vi "RunTest.vi"(8 "error in (no error)":errorcluster, 11 "Prueba07 in":refnum<class "Prueba07.lvclass">) -> (0 "error out":errorcluster, 2 "resultado":string, 3 "Prueba07 out":refnum<class "Prueba07.lvclass">)   [LabVIEW 2019, in "Prueba07.lvclass"]
uses:
  Prueba07.lvclass
  Prueba04/Control/Slide.ctl
  Prueba07.lvclass/Prueba07.ctl
  ClusterGEN.ctl
  Controles/MessageP07.ctl
  Controles/EstadosP07.ctl
  <vilib>/Utility/error.llb/DialogType.ctl
  QMH/Message Queue/Enqueue Message (Single).vi
  <vilib>/Utility/error.llb/Error Cluster From Error Code.vi
  <vilib>/ErrorRing/Error Ring.xnode
  <vilib>/Utility/miscctls.llb/LVRowAndColumnTypeDef.ctl
  Prueba/Prueba.lvclass
  Prueba04/Prueba04.lvclass
  QMH/User Event - Stop/User Event - Stop.lvlib
  QMH/Message Queue/Message Queue.lvlib
panel:
  out "GEN":string
  out "n°filas":i32
  out "Vref_NivMax":dbl[](array[numeric])
  out "tablaRef (Num)":dbl[](array[numeric])
  out "Pict Ring 2":u16(ring)
  out "Pict Ring 3":u16(ring)
  out "cumple_no_cumple":bool
  out "Vref":dbl
  in  "Tab":enum32{"Page 1", "Page 2"}(tab)
  out "frecuencia1":dbl=140.0
  out "nivelRef":dbl=95.0 format="%.1f"
  in  "guardar_Vref":bool
  in  "generar1":bool
  in  "AjusteAmp":T1=50.0 caption="Ajuste de amplitud [mV]" scale=0.0..100.0
  out "voltaje1":dbl format="%.1f"
  out "frecuencia1":dbl format="%.1f"
  in  "seguir":bool
  out "Pict Ring 1":u16(ring)
  out "Pict Ring":u16(ring)
  out "RefActual":string
  in  "generarNivMax":bool caption="PruebaSup"
  in  "generarNivRef":bool caption="PruebaSup"
  in  "Tabla":string[][](table)
  in  "salir":bool
  out "cumple":bool
  out "no_cumple":bool
  out "voltaje2":dbl format="%.1f"
  out "frecuencia2":dbl format="%#.1f"
  out "RangoRefActual":string
  # "Elección Señal de Referencia\nsegún marca y modelo de sonómetro"
  # "Nivel Señal Referencia"
  # "Frecuencia"
  # "Monitoreo"
  # "Frecuencia"
  # "Hz"
  # "Voltaje"
  # "mV"
  # "7. Linealidad de nivel incluyendo el control de rangos de niveles. IEC 61672-3: 2006 Cláusula 15"
  # "Tabla Resultados"
  # "Nivel de Referencia"
  # "Nivel Max Rn - 5 db(A)"
  # "Rango dB"
  # "Referencia dB"
  # "Cumple"
  # "No Cumple"
  # "7. Linealidad de nivel incluyendo el control de rangos de niveles. IEC 61672-3: 2006 Cláusula 15"
  # "Monitoreo"
  # "Frecuencia"
  # "Hz"
  # "Voltaje"
  # "mV"
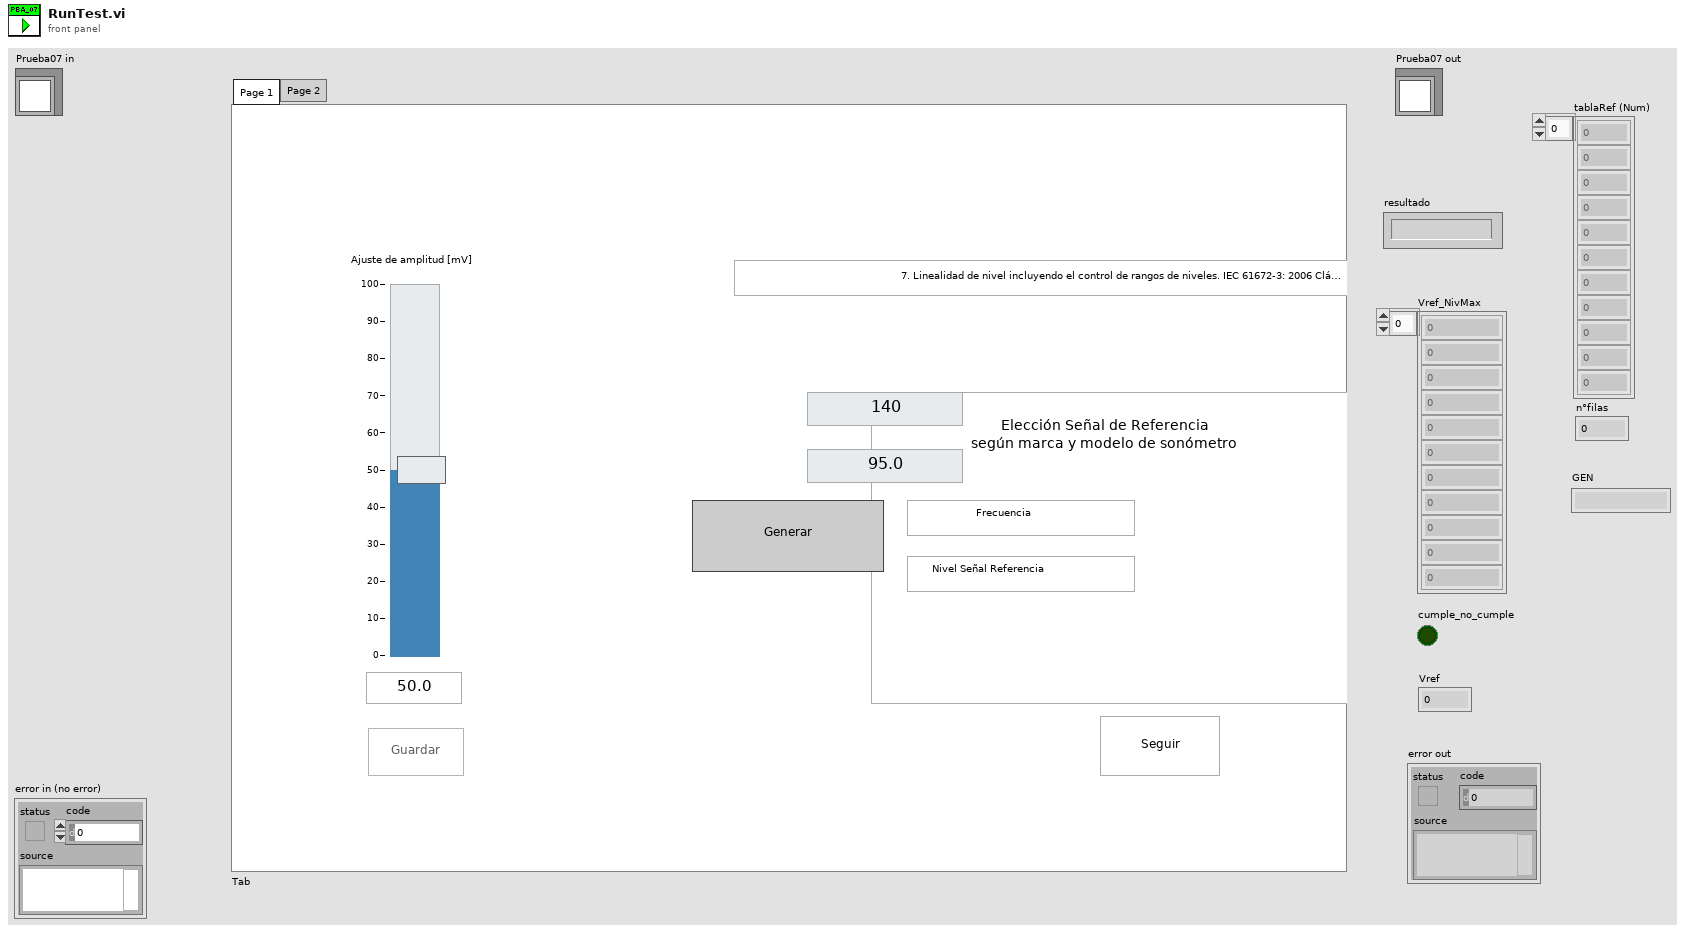
[diagram p1: front panel]
types:
  T1 = typedef "Prueba04.lvclass/Slide.ctl" = dbl
  T2 = typedef "LVRowAndColumnTypeDef.ctl" = cluster{"Row":i32, "Column":i32}
  T3 = typedef "Message Queue.lvlib/All Message Queues.ctl" = cluster{"MHL":refnum<queue>, "Inst_CNT90":refnum<queue>, "Inst_DS360":refnum<queue>, "Inst_Keithley2002":refnum<queue>, "Inst_DAQ":refnum<queue>, "BD":refnum<queue>, "Pistofono":refnum<queue>, "Nexus":refnum<queue>}
  T4 = enum32{"Page 1", "Page 2", "Page 3", "Page 4", "Page 5", "Page 6", "Page 7"}
  T5 = typedef "Prueba07.lvclass/ClusterGEN.ctl" = cluster{"frec":dbl, "amp":dbl}
  T6 = enum8{"Enabled", "Disabled", "Disabled and Grayed Out"}
  T7 = cluster{"ControlName":string, "ControlReference":refnum<vi>}[]
  T8 = typedef "Prueba07.lvclass/MessageP07.ctl" = cluster{"Estados":T9, "Data":variant}
  T9 = typedef "Prueba07.lvclass/EstadosP07.ctl" = enum16{"inicio", "LeerArchivoConfiguracion", "InicializarInstrumentos", "DetieneInstrumentos", "leerRangosdB", "configuraTabla", "FrecAmp1", "FrecAmp2_Vref", "updateUI", "FrecAmp2_Vref_NivMax", "iniciarGEN", "detenerGEN", "guardaVref", "monitoreo", "calcular_Vref", "guardarMedicionesNivRef", "guardarMedicionesNivMax", "ingresaMediciones", "cumplimiento", "listo_evaluar", "evaluar", "final", "salir"}
  T10 = typedef "DialogType.ctl" = u16
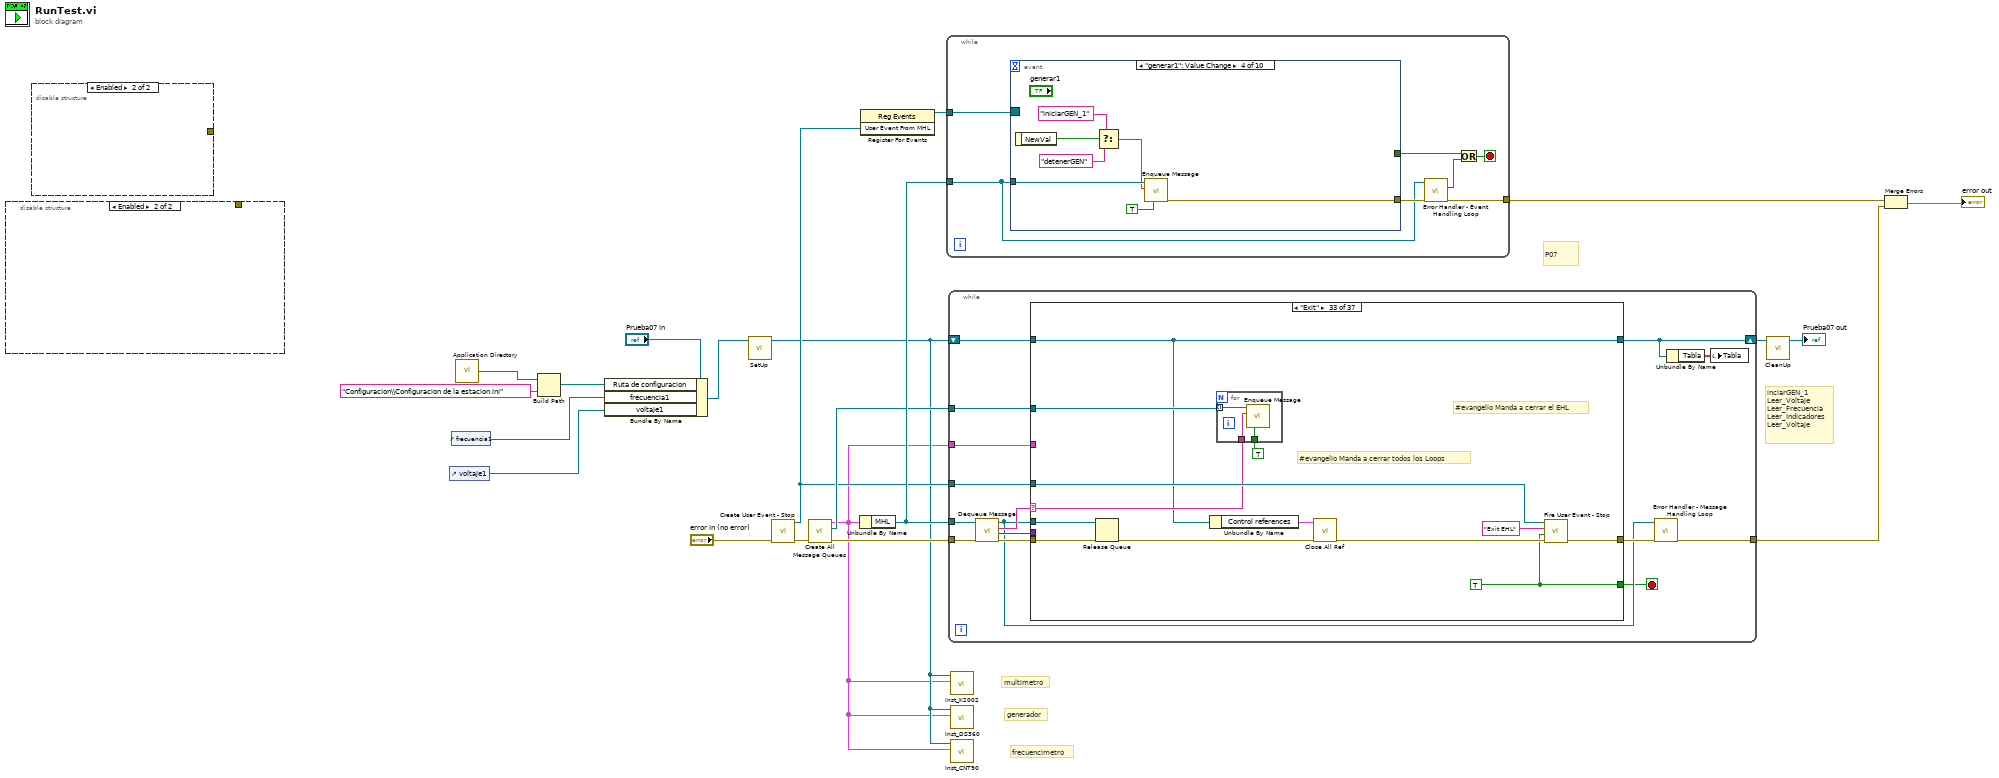
[diagram p0: block diagram]
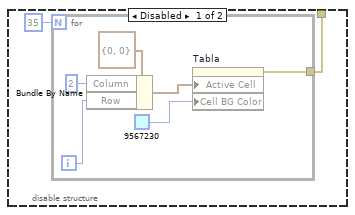
[diagram p2: hidden frame]
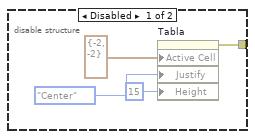
[diagram p3: hidden frame]
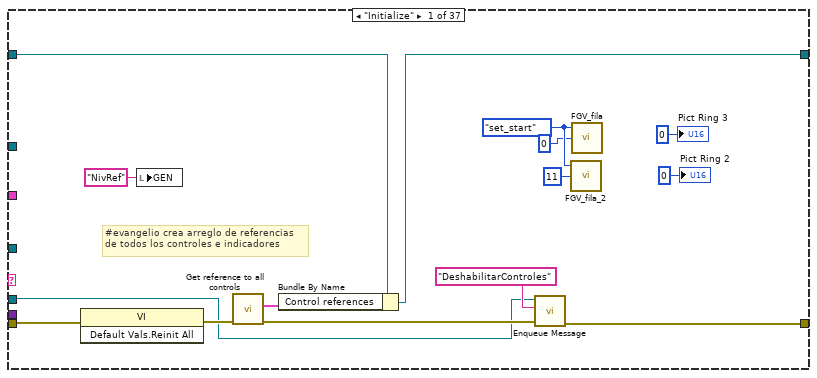
[diagram p4: hidden frame]
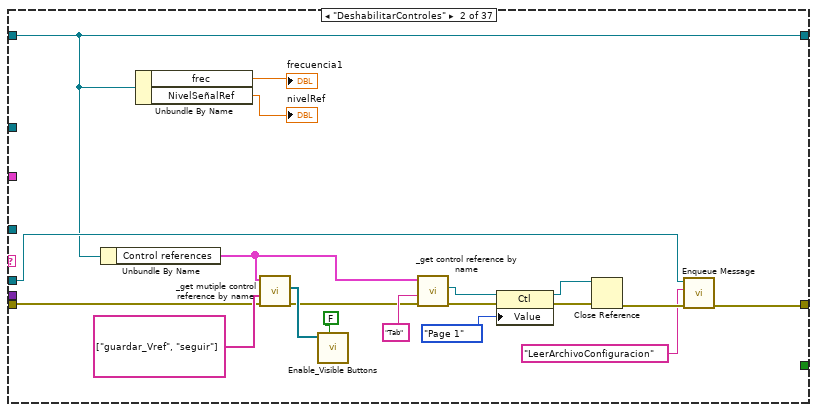
[diagram p5: hidden frame]
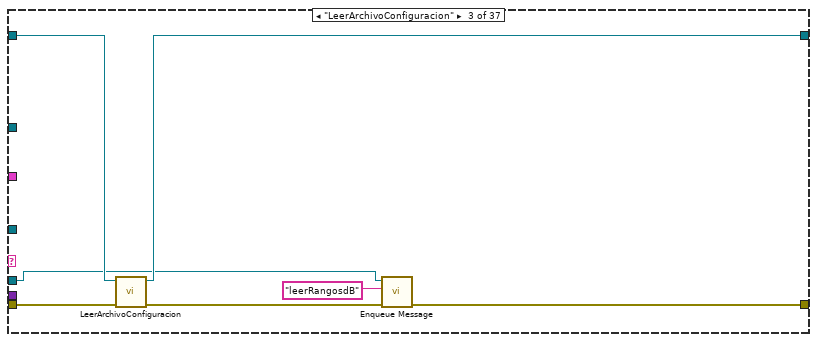
[diagram p6: hidden frame]
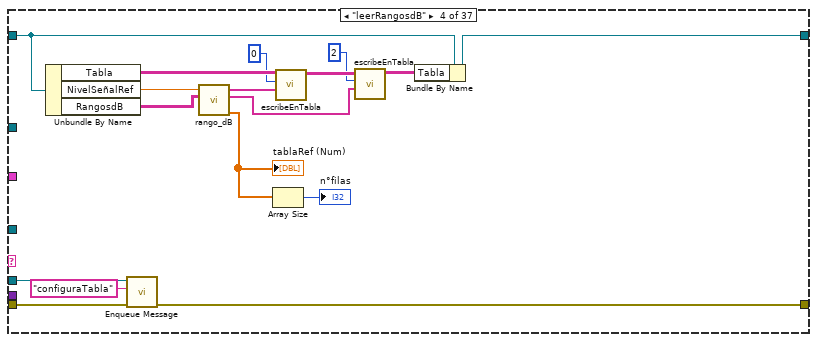
[diagram p7: hidden frame]
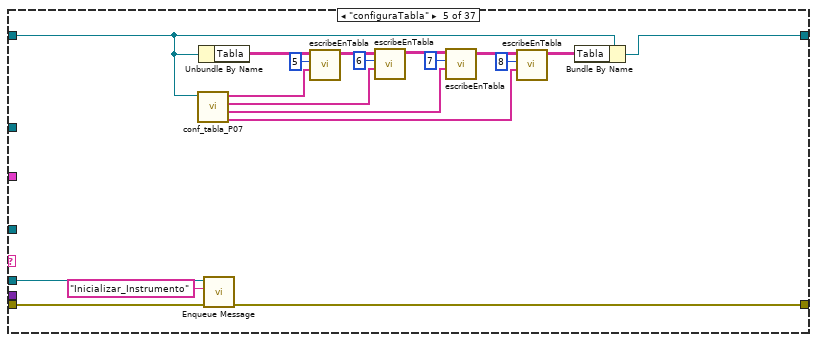
[diagram p8: hidden frame]
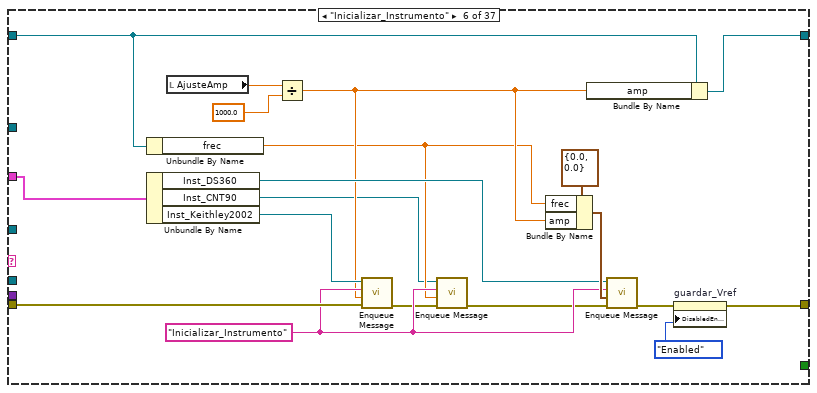
[diagram p9: hidden frame]
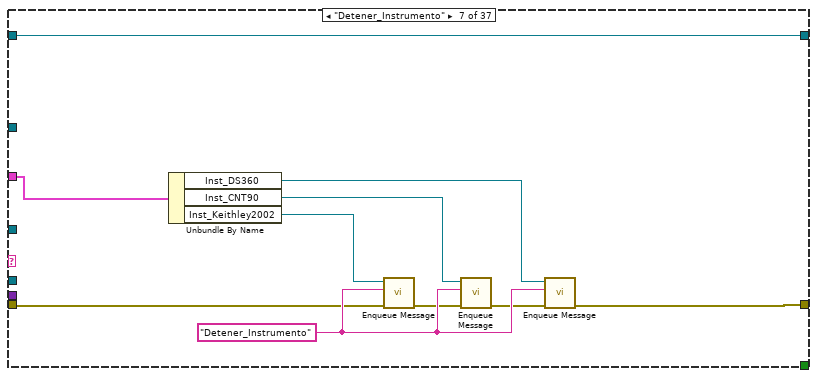
[diagram p10: hidden frame]
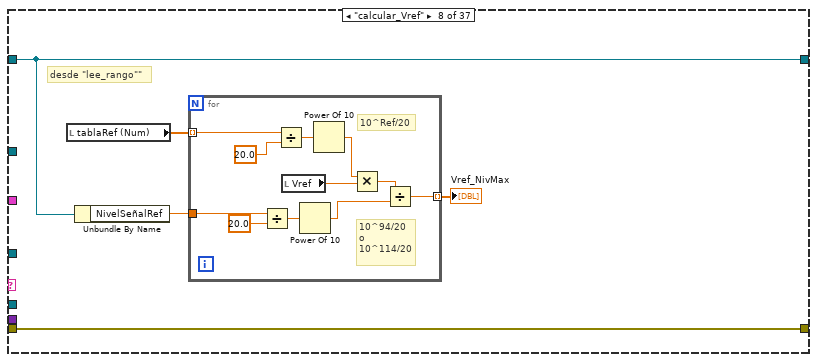
[diagram p11: hidden frame]
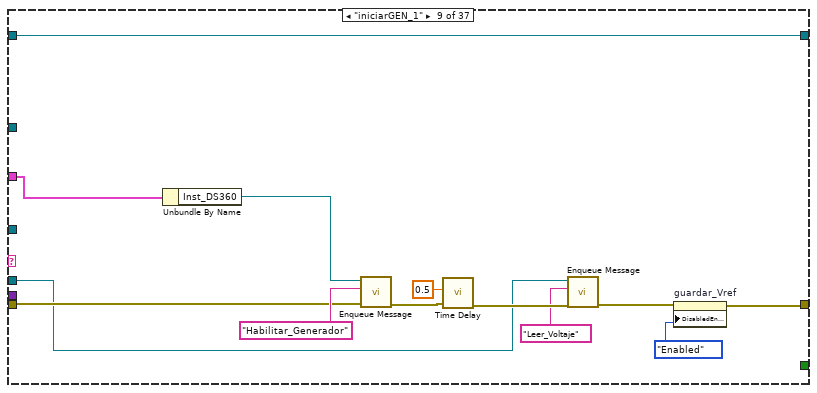
[diagram p12: hidden frame]
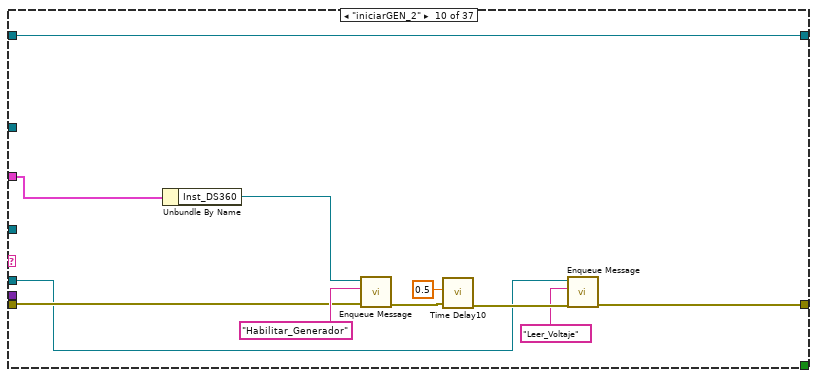
[diagram p13: hidden frame]
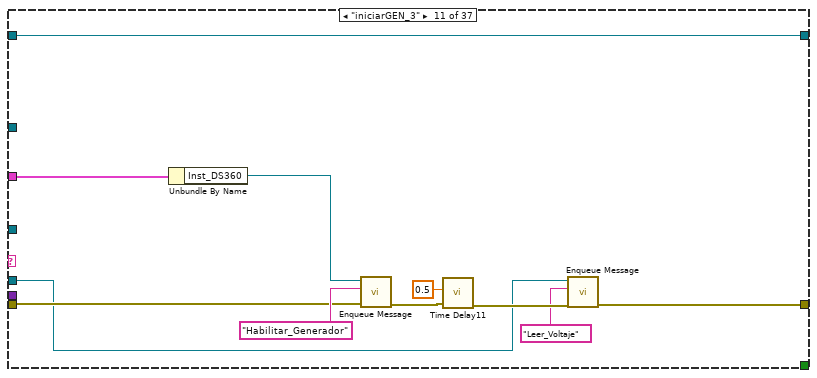
[diagram p14: hidden frame]
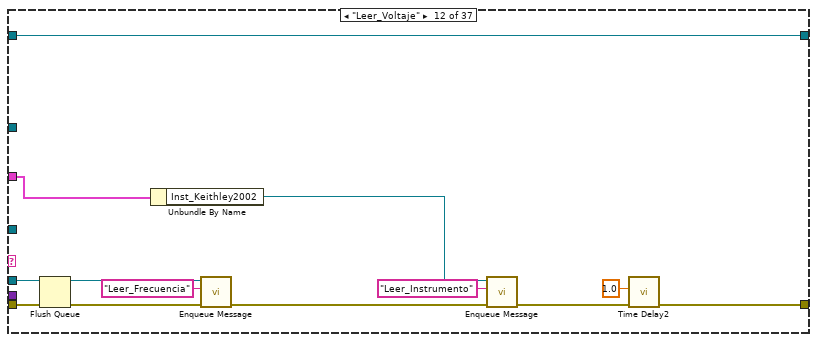
[diagram p15: hidden frame]
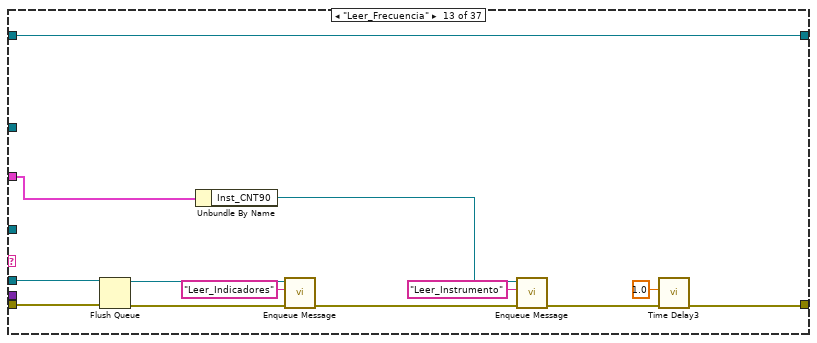
[diagram p16: hidden frame]
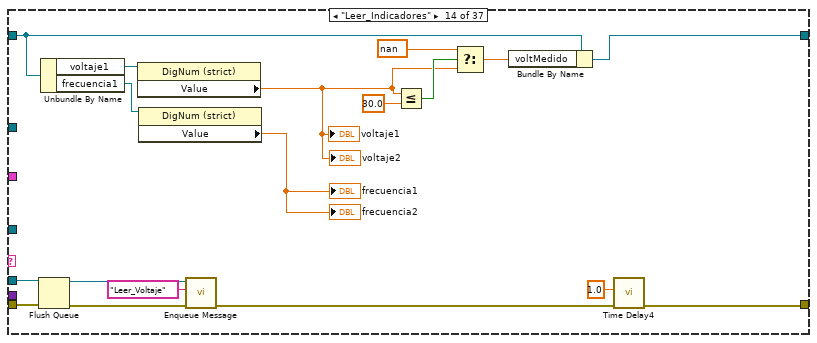
[diagram p17: hidden frame]
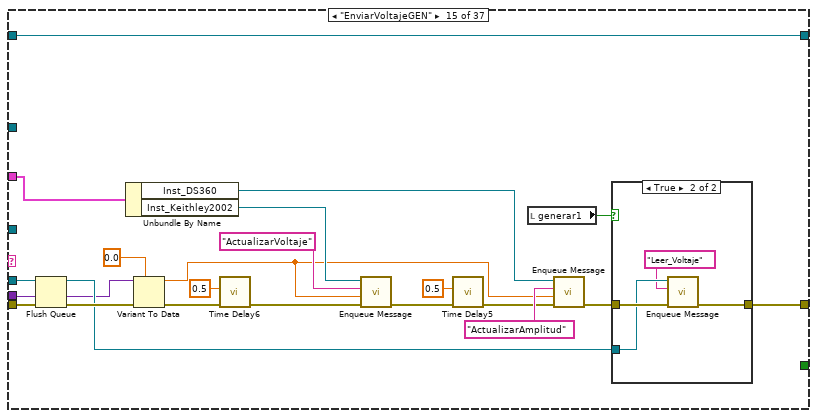
[diagram p18: hidden frame]
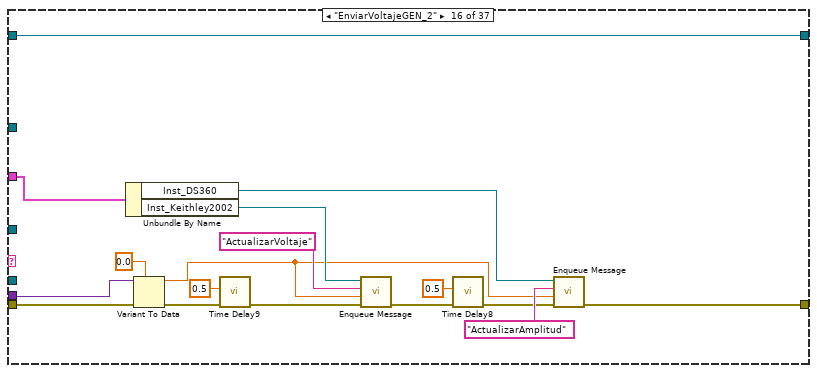
[diagram p20: hidden frame]
diagram:
  # "inciarGEN_1\nLeer_Voltaje\nLeer_Frecuencia\nLeer_Indicadores\nLeer_Voltaje"
  # "P07"
  # "frecuencimetro"
  # "generador"
  # "multimetro"
  n1 = disable-structure shown="Enabled" {
    disable-tunnel: [w23 _] -> _
    frame Disabled {
      n2 = for {
        N: 35 -> [_]
        tunnel: [w25] -> w23
        i -> [w24]
        n3 = Bundle By Name(cluster=T2 {"Row"=0, "Column"=0} ("Active Cell:Active Cell"), "Column"=2, "Row"=w24) -> (w27:T2)
        n4 = property on="Tabla" class="Tbl (strict)"("Active Cell"=w27, "Cell BG Color"=u32 9567230) -> (error out=w25:errorcluster)  [unwired: 2 in, 1 out]
      }
    }
    frame Enabled {
    }
  }
  n5 = disable-structure shown="Enabled" {
    disable-tunnel: [w32 _] -> _
    frame Disabled {
      n6 = property on="Tabla" class="Tbl (strict)"("Active Cell"=T2 {"Row"=-2, "Column"=-2} ("Active Cell:Active Cell"), "Justify"=enum16{"Left", "Center", "Right"}."Center" ("Active Cell:Cell Justification"), "Height"=u32 15 ("Active Cell:Cell Font:Size")) -> (error out=w32:errorcluster)  [unwired: 2 in, 1 out]
    }
    frame Enabled {
    }
  }
  n7 = control-ref of="voltaje1"() -> (w3:refnum<vi>)
  n8 = control-ref of="frecuencia1"() -> (w4:refnum<vi>)
  n9 = call <vilib>:"Application Directory.vi"() -> ("Application Directory"=w17:path)
  n10 = Build Path(base path=w17, name or relative path="Configuracion\\Configuracion de la estacion.ini") -> (appended path=w16:path)
  n11 = Bundle By Name(cluster="Prueba07 in", "Ruta de configuracion"=w16, "frecuencia1"=w4, "voltaje1"=w3) -> (w14:refnum<class "Prueba07.lvclass">)
  n12 = call-dynamic "SetUp.vi"("Prueba07 in"=w14) -> ("Prueba07 out"=w6:refnum<class "Prueba07.lvclass">)  [unwired: 9 in, 1 out]
  n13 = call "Create User Event - Stop.vi"("error in (no error)"="error in (no error)") -> ("error out"=w13:errorcluster, "User Event From MHL"=w8:refnum<user-event>)  [unwired: 9 in]
  n14 = call "Create All Message Queues.vi"("error in (no error)"=w13) -> ("error out"=w11:errorcluster, "PL Queues Array"=w9:refnum<queue>[], "All Message Queues out"=w5:T3)  [unwired: 8 in]
  n15 = Unbundle By Name(w5) -> ("MHL"=w10:refnum<queue>)
  n16 = register-events(w8) -> (reference out=w7:refnum<event-registration>)  [unwired: 2 in, 1 out]
  n17 = while {
    tunnel: w10 -> [w36]
    tunnel: [w38] -> w21
    tunnel: w7 -> [w35]
    stop <- w40 stop-if-true
    n18 = event shown="[3] \"generar1\": Value Change" {
      selector: w35 -> [_ _ _ _ _ _ _ _ _ _]
      dyn-events: _ -> [_ _ _ _ _ _ _ _ _ _]
      timeout: _ -> [_ _ _ _ _ _ _ _ _ _]
      tunnel: w36 -> [w43 _ w54 w61 w68 w75 w81 w87 w91 w97]
      tunnel: [w46 _ _ w62 w69 w76 w78 w88 w92 w96] -> w39
      tunnel: [_ w47 _ _ _ _ _ _ _ _] -> w34
      event "salir": Value Change {
        n19 = event-data() -> ()  [unwired: 1 in, 1 out]
        n20 = call-poly "Enqueue Message.vi"("Message"="Detener_Instrumento", "Message Queue"=w43) -> ("error out"=w41:errorcluster, "dup Message Queue"=w42:refnum<queue>)  [unwired: 8 in]
        n21 = call-poly "Enqueue Message.vi"("error in (no error)"=w41, "Message"="Exit", "Message Queue"=w42) -> ("error out"=w46:errorcluster)  [unwired: 7 in, 1 out]
      }
      event User Event {
        n22 = event-data() -> ("User Event"=w49:string, "Event Data"=w48:variant)  [unwired: 1 in]
        n23 = case shown="\"Exit EHL\"" w49 {
          tunnel: w48 -> [_ w51]
          tunnel: [_ w50] -> w47
          frame Default {
          }
          frame "Exit EHL" {
            # "#evangelio Termina\nla ejecucion del EHL"
            n24 = Variant To Data(type=TRUE, Variant=w51) -> (data=w50:bool)  [unwired: 1 in, 1 out]
          }
        }
      }
      event Panel Close? {
        w53 = TRUE
        n25 = event-data() -> ()  [unwired: 1 in, 1 out]
        n26 = call-poly "Enqueue Message.vi"("Priority Message? (F)"=w53, "Message"="Confirmar Salida", "Message Queue"=w54) -> ()  [unwired: 7 in, 2 out]
        n27 = event-data("Discard?"=w53) -> ()  [unwired: 1 in, 1 out]
      }
      event "generar1": Value Change {
        n28 = event-data() -> ("NewVal"=w60:bool)  [unwired: 1 in]
        n29 = Select(t="iniciarGEN_1" ("Message"), s=w60, f="detenerGEN" ("Message")) -> (s? t:f=w57:string)
        n30 = call-poly "Enqueue Message.vi"("Priority Message? (F)"=TRUE, "Message"=w57, "Message Queue"=w61) -> ("error out"=w62:errorcluster)  [unwired: 7 in, 1 out]
      }
      event "generarNivRef": Value Change {
        n31 = event-data() -> ("NewVal"=w67:bool)  [unwired: 1 in]
        n32 = Select(t="FrecAmp2_Vref", s=w67, f="guardarMedicionesNivRef") -> (s? t:f=w64:string)
        n33 = call-poly "Enqueue Message.vi"("Priority Message? (F)"=TRUE, "Message"=w64, "Message Queue"=w68) -> ("error out"=w69:errorcluster)  [unwired: 7 in, 1 out]
      }
      event "generarNivMax": Value Change {
        n34 = event-data() -> ("NewVal"=w74:bool)  [unwired: 1 in]
        n35 = Select(t="FrecAmp2_Vref_NivMax", s=w74, f="guardarMedicionesNivMax") -> (s? t:f=w71:string)
        n36 = call-poly "Enqueue Message.vi"("Priority Message? (F)"=TRUE, "Message"=w71, "Message Queue"=w75) -> ("error out"=w76:errorcluster)  [unwired: 7 in, 1 out]
      }
      event "seguir": Value Change {
        n37 = event-data() -> ()  [unwired: 1 in, 1 out]
        n38 = call-poly "Enqueue Message.vi"("Message"="calcular_Vref", "Message Queue"=w81) -> ("error out"=w79:errorcluster)  [unwired: 8 in, 1 out]
        n39 = property on="Tab" class="TabCtl (strict)"(error in=w79, "Value"=enum32{"Page 1", "Page 2"}."Page 2" ("Tab")) -> (error out=w78:errorcluster)  [unwired: 1 in, 1 out]
      }
      event Value Change {
        n40 = event-data() -> ()  [unwired: 1 in, 1 out]
        n41 = Divide(x="AjusteAmp", y=T1 1000.0) -> (x/y=w83:T1)
        n42 = call-poly "Enqueue Message.vi"("Priority Message? (F)"=TRUE, "Message Data"=w83, "Message"="EnviarVoltajeGEN", "Message Queue"=w87) -> ("error out"=w88:errorcluster)  [unwired: 6 in, 1 out]
      }
      event "guardar_Vref": Value Change {
        n43 = event-data() -> ()  [unwired: 1 in, 1 out]
        n44 = call-poly "Enqueue Message.vi"("Priority Message? (F)"=TRUE, "Message"="guardarVref", "Message Queue"=w91) -> ("error out"=w92:errorcluster)  [unwired: 7 in, 1 out]
      }
      event "Tabla": Value Change {
        n45 = event-data() -> ("NewVal"=w95:string[][])  [unwired: 1 in]
        n46 = call-poly "Enqueue Message.vi"("Priority Message? (F)"=TRUE, "Message Data"=w95, "Message"="ingresaMediciones", "Message Queue"=w97) -> ("error out"=w96:errorcluster)  [unwired: 6 in, 1 out]
      }
    }
    n47 = call "Error Handler - Event Handling Loop.vi"("error in (no error)"=w39, "Message Queue"=w36) -> ("dup error in"=w38:errorcluster, "Error?"=w37:bool)  [unwired: 7 in, 1 out]
    n48 = Or(x=w34, y=w37) -> (x .or. y?=w40:bool)
  }
  n49 = while {
    tunnel: w10 -> [w108]
    tunnel: w11 -> [w109]
    tunnel: [w100] -> w20
    shift-right: [w111] -> w2
    shift-left: w6 -> [w112]
    tunnel: w5 -> [w104]
    tunnel: w9 -> [w103]
    tunnel: w8 -> [w102]
    stop <- w98 stop-if-true
    n50 = call "Dequeue Message.vi"("error in (no error)"=w109, "Message Queue"=w108) -> ("error out"=w107:errorcluster, "Message Data"=w106:variant, "Message"=w105:string, "dup Message Queue"=w99:refnum<queue>)  [unwired: 6 in]
    n51 = case shown="\"Exit\"" w105 {
      selector: w105 -> [_ _ _ _ _ _ _ _ _ _ _ _ _ _ _ _ _ _ _ _ _ _ _ _ _ _ _ _ _ _ _ _ w645 _ w676 _ _]
      tunnel: w106 -> [_ _ _ _ _ _ _ _ _ _ _ _ _ _ w317 w343 w360 _ _ _ _ w489 _ _ _ _ _ w602 w607 _ _ _ _ _ _ w687 _]
      tunnel: w107 -> [w123 w133 w153 w169 w183 w208 w212 w219 w238 w251 w262 w274 w287 w308 w321 w348 w365 w396 w425 w452 w484 w501 w508 w529 w570 w579 w595 w604 w609 w617 w630 w640 w649 w661 _ w692 w695]
      tunnel: [w121 w131 w149 w158 w173 w193 w210 w219 w246 w248 w259 w272 w286 w306 w318 w344 w361 w395 w408 w426 w458 w499 w506 w528 w568 w579 w595 w601 w606 w614 w631 w640 w642 w659 w675 w690 w695] -> w101
      tunnel: [_ _ _ _ _ _ _ _ _ _ _ _ _ _ _ _ _ _ _ _ _ _ _ _ _ _ _ _ _ _ _ _ w643 _ _ _ _] -> w98
      tunnel: w99 -> [w122 w132 w148 w157 w172 _ _ _ w236 w249 w260 w270 w284 w307 w320 _ _ w393 w424 w451 w483 w496 w505 w527 w569 _ _ _ _ w616 _ _ w648 w660 _ w691 _]
      tunnel: w112 -> [w119 w128 w152 w170 w180 w192 w209 w222 w245 w258 w269 w271 w283 w300 w335 w357 w374 w381 w399 w428 w457 w491 w504 w520 w563 w580 w594 w603 w608 w613 w633 w641 w644 w658 w674 w689 w694]
      tunnel: [w120 w128 w151 w166 w182 w207 w209 w222 w245 w258 w269 w271 w283 w301 w335 w357 w374 w391 w422 w447 w479 w490 w503 w520 w563 w580 w594 w603 w608 w613 w633 w641 w644 w658 w674 w689 w694] -> w111
      tunnel: w104 -> [_ _ _ _ _ w197 w211 _ w237 w250 w261 w273 w285 _ w319 w345 w362 _ _ _ _ _ _ _ _ _ _ _ _ w615 _ _ _ _ _ _ _]
      tunnel: w103 -> [_ _ _ _ _ _ _ _ _ _ _ _ _ _ _ _ _ _ _ _ _ _ _ _ _ _ _ _ _ _ _ _ w647 _ _ _ _]
      tunnel: w102 -> [_ _ _ _ _ _ _ _ _ _ _ _ _ _ _ _ _ _ _ _ _ _ _ _ _ _ _ _ _ _ _ _ w646 _ _ _ _]
      frame "Initialize" {
        w117 = enum16{"increment", "set_start", "get"}."set_start" ("action")
        # "#evangelio crea arreglo de referencias\nde todos los controles e indicadores"
        n52 = invoke class="VI" method="Default Vals.Reinit All"(error in=w123) -> (error out=w126:errorcluster)  [unwired: 2 in, 2 out]
        n53 = local write "GEN"("NivRef" ("GEN")) -> ()
        n54 = call "Get reference to all controls.vi"("error in (no error)"=w126) -> ("error out"=w124:errorcluster, "Control references"=w125:T7)  [unwired: 5 in]
        n55 = Bundle By Name(cluster=w119, "Control references"=w125) -> (w120:refnum<class "Prueba07.lvclass">)
        n56 = call-poly "Enqueue Message.vi"("error in (no error)"=w124, "Message"="DeshabilitarControles", "Message Queue"=w122) -> ("error out"=w121:errorcluster)  [unwired: 7 in, 1 out]
        n57 = call "FGV_fila_2.vi"("fila_inicial"=11, "action"=w117) -> ()  [unwired: 2 in, 2 out]
        n58 = call "FGV_fila.vi"("fila_inicial"=0, "action"=w117) -> ()  [unwired: 2 in, 2 out]
        "Pict Ring 2" <- u16 0 ("Pict Ring 2")
        "Pict Ring 3" <- u16 0 ("Pict Ring 3")
      }
      frame "DeshabilitarControles" {
        n59 = Unbundle By Name(w128) -> ("Control references"=w142:T7)
        n60 = Unbundle By Name(w128) -> ("frec"=→"frecuencia1":dbl, "NivelSeñalRef"=→"nivelRef":dbl)
        n61 = call "_get mutiple control reference by name.vi"("error in (no error)"=w133, "Control names"=string[] ["guardar_Vref", "seguir"], "Control references"=w142) -> ("error out"=w139:errorcluster, "References"=w140:refnum<vi>[])  [unwired: 3 in]
        n62 = call "Enable_Visible Buttons.vi"("Enable? (T)"=FALSE, "Controls Ref Array"=w140) -> ()  [unwired: 10 in]
        n63 = call "_get control reference by name.vi"("error in (no error)"=w139, "Control name"="Tab" ("Message"), "Control references"=w142) -> ("error out"=w146:errorcluster, "Ctl Refnum"=w144:refnum<vi>)  [unwired: 3 in]
        n64 = property class="Ctl"(reference=w144, error in=w146, "Value"=T4."Page 1" ("Tab_Prueba04")) -> (reference out=w135:refnum<vi>, error out=w137:errorcluster)
        n65 = Close Reference(reference=w135, error in (no error)=w137) -> (error out=w136:errorcluster)
        n66 = call-poly "Enqueue Message.vi"("error in (no error)"=w136, "Message"="LeerArchivoConfiguracion", "Message Queue"=w132) -> ("error out"=w131:errorcluster)  [unwired: 7 in, 1 out]
      }
      frame "LeerArchivoConfiguracion" {
        n67 = call "LeerArchivoConfiguracion.vi"("error in"=w153, "Prueba07 in"=w152) -> ("error out"=w150:errorcluster, "Prueba07 out"=w151:refnum<class "Prueba07.lvclass">)  [unwired: 8 in]
        n68 = call-poly "Enqueue Message.vi"("error in (no error)"=w150, "Message"="leerRangosdB", "Message Queue"=w148) -> ("error out"=w149:errorcluster)  [unwired: 7 in, 1 out]
      }
      frame "leerRangosdB" {
        n69 = Unbundle By Name(w170) -> ("Tabla"=w165:string[][], "NivelSeñalRef"=w168:dbl, "RangosdB"=w167:string[][])
        n70 = call-poly "Enqueue Message.vi"("error in (no error)"=w169, "Message"="configuraTabla", "Message Queue"=w157) -> ("error out"=w158:errorcluster)  [unwired: 7 in, 1 out]
        n71 = call "rango_dB.vi"("rangosDB in"=w167, "referencia[dB]"=w168) -> ("tablaRef (Num)"=w156:dbl[], "Referencia[dB]"=w159:string[], "rango[dB]"=w160:string[])  [unwired: 7 in]
        "tablaRef (Num)" <- w156
        n72 = Array Size(array=w156) -> (size(s)=→"n°filas":i32)
        n73 = call "escribeEnTabla.vi"("parametros"=w160, "col"=0, "tabla in"=w165) -> ("tabla out"=w164:string[][])  [unwired: 8 in]
        n74 = call "escribeEnTabla.vi"("parametros"=w159, "col"=2, "tabla in"=w164) -> ("tabla out"=w163:string[][])  [unwired: 8 in]
        n75 = Bundle By Name(cluster=w170, "Tabla"=w163) -> (w166:refnum<class "Prueba07.lvclass">)
      }
      frame "configuraTabla" {
        n76 = call "conf_tabla_P07.vi"("Prueba07 out"=w180) -> ("cumplimiento"=w174:string[], "Tol -"=w177:string[], "Tol +"=w178:string[], "incertidumbre"=w179:string[])  [unwired: 7 in]
        n77 = Unbundle By Name(w180) -> ("Tabla"=w181:string[][])
        n78 = call-poly "Enqueue Message.vi"("error in (no error)"=w183, "Message"="Inicializar_Instrumento", "Message Queue"=w172) -> ("error out"=w173:errorcluster)  [unwired: 7 in, 1 out]
        n79 = call "escribeEnTabla.vi"("parametros"=w179, "col"=5, "tabla in"=w181) -> ("tabla out"=w189:string[][])  [unwired: 8 in]
        n80 = call "escribeEnTabla.vi"("parametros"=w178, "col"=6, "tabla in"=w189) -> ("tabla out"=w188:string[][])  [unwired: 8 in]
        n81 = call "escribeEnTabla.vi"("parametros"=w177, "col"=7, "tabla in"=w188) -> ("tabla out"=w184:string[][])  [unwired: 8 in]
        n82 = call "escribeEnTabla.vi"("parametros"=w174, "col"=8, "tabla in"=w184) -> ("tabla out"=w176:string[][])  [unwired: 8 in]
        n83 = Bundle By Name(cluster=w180, "Tabla"=w176) -> (w182:refnum<class "Prueba07.lvclass">)
      }
      frame "Inicializar_Instrumento" {
        w202 = "Inicializar_Instrumento" ("Message")
        n84 = Unbundle By Name(w192) -> ("frec"=w191:dbl)
        n85 = Unbundle By Name(w197) -> ("Inst_DS360"=w195:refnum<queue>, "Inst_CNT90"=w190:refnum<queue>, "Inst_Keithley2002"=w204:refnum<queue>)
        n86 = local read "AjusteAmp"() -> (w206:T1)
        n87 = Divide(x=w206, y=T1 1000.0) -> (x/y=w194:T1)
        n88 = call-poly "Enqueue Message.vi"("error in (no error)"=w208, "Message Data"=w194, "Message"=w202, "Message Queue"=w204) -> ("error out"=w201:errorcluster)  [unwired: 6 in, 1 out]
        n89 = call-poly "Enqueue Message.vi"("error in (no error)"=w201, "Message Data"=w191, "Message"=w202, "Message Queue"=w190) -> ("error out"=w200:errorcluster)  [unwired: 6 in, 1 out]
        n90 = Bundle By Name(cluster=T5 {"frec"=0.0, "amp"=0.0} ("clusterGEN"), "frec"=w191, "amp"=w194) -> (w203:T5)
        n91 = Bundle By Name(cluster=w192, "amp"=w194) -> (w207:refnum<class "Prueba07.lvclass">)
        n92 = call-poly "Enqueue Message.vi"("error in (no error)"=w200, "Message Data"=w203, "Message"=w202, "Message Queue"=w195) -> ("error out"=w198:errorcluster)  [unwired: 6 in, 1 out]
        n93 = property on="guardar_Vref" class="Bool"(error in=w198, "DisabledEnum"=T6."Enabled" ("Disabled")) -> (error out=w193:errorcluster)  [unwired: 1 in, 1 out]
      }
      frame "Detener_Instrumento" {
        w215 = "Detener_Instrumento" ("Message")
        n94 = Unbundle By Name(w211) -> ("Inst_DS360"=w218:refnum<queue>, "Inst_CNT90"=w217:refnum<queue>, "Inst_Keithley2002"=w216:refnum<queue>)
        n95 = call-poly "Enqueue Message.vi"("error in (no error)"=w212, "Message"=w215, "Message Queue"=w216) -> ("error out"=w214:errorcluster)  [unwired: 7 in, 1 out]
        n96 = call-poly "Enqueue Message.vi"("error in (no error)"=w214, "Message"=w215, "Message Queue"=w217) -> ("error out"=w213:errorcluster)  [unwired: 7 in, 1 out]
        n97 = call-poly "Enqueue Message.vi"("error in (no error)"=w213, "Message"=w215, "Message Queue"=w218) -> ("error out"=w210:errorcluster)  [unwired: 7 in, 1 out]
      }
      frame "calcular_Vref" {
        # "desde \"lee_rango\"\""
        n98 = local read "tablaRef (Num)"() -> (w221:dbl[])
        n99 = Unbundle By Name(w222) -> ("NivelSeñalRef"=w223:dbl)
        n100 = for {
          tunnel: w223 -> [w229]
          tunnel: [w226] -> w220 mode=indexing
          tunnel: w221 -> [w224] mode=indexing
          # "10^94/20\no \n10^114/20"
          # "10^Ref/20"
          n101 = Divide(x=w229, y=20.0) -> (x/y=w230:dbl)
          n102 = Divide(x=w224, y=20.0) -> (x/y=w233:dbl)
          n103 = local read "Vref"() -> (w225:dbl)
          n104 = Power Of 10(x=w230) -> (10^x=w227:dbl)
          n105 = Power Of 10(x=w233) -> (10^x=w232:dbl)
          n106 = Multiply(x=w232, y=w225) -> (x*y=w231:dbl)
          n107 = Divide(x=w231, y=w227) -> (x/y=w226:dbl)
        }
        "Vref_NivMax" <- w220
      }
      frame "iniciarGEN_1" {
        n108 = Unbundle By Name(w237) -> ("Inst_DS360"=w243:refnum<queue>)
        n109 = call-poly "Enqueue Message.vi"("error in (no error)"=w238, "Message"="Habilitar_Generador", "Message Queue"=w243) -> ("error out"=w241:errorcluster)  [unwired: 7 in, 1 out]
        n110 = call "Time Delay"("error in (no error)"=w241, "Delay Time (s)"=0.5) -> ("error out"=w240:errorcluster)  [unwired: 9 in]
        n111 = call-poly "Enqueue Message.vi"("error in (no error)"=w240, "Message"="Leer_Voltaje", "Message Queue"=w236) -> ("error out"=w235:errorcluster)  [unwired: 7 in, 1 out]
        n112 = property on="guardar_Vref" class="Bool"(error in=w235, "DisabledEnum"=T6."Enabled" ("Disabled")) -> (error out=w246:errorcluster)  [unwired: 1 in, 1 out]
      }
      frame "iniciarGEN_2" {
        n113 = Unbundle By Name(w250) -> ("Inst_DS360"=w256:refnum<queue>)
        n114 = call-poly "Enqueue Message.vi"("error in (no error)"=w251, "Message"="Habilitar_Generador", "Message Queue"=w256) -> ("error out"=w254:errorcluster)  [unwired: 7 in, 1 out]
        n115 = call "Time Delay10"("error in (no error)"=w254, "Delay Time (s)"=0.5) -> ("error out"=w253:errorcluster)  [unwired: 9 in]
        n116 = call-poly "Enqueue Message.vi"("error in (no error)"=w253, "Message"="Leer_Voltaje", "Message Queue"=w249) -> ("error out"=w248:errorcluster)  [unwired: 7 in, 1 out]
      }
      frame "iniciarGEN_3" {
        n117 = Unbundle By Name(w261) -> ("Inst_DS360"=w267:refnum<queue>)
        n118 = call-poly "Enqueue Message.vi"("error in (no error)"=w262, "Message"="Habilitar_Generador", "Message Queue"=w267) -> ("error out"=w265:errorcluster)  [unwired: 7 in, 1 out]
        n119 = call "Time Delay11"("error in (no error)"=w265, "Delay Time (s)"=0.5) -> ("error out"=w264:errorcluster)  [unwired: 9 in]
        n120 = call-poly "Enqueue Message.vi"("error in (no error)"=w264, "Message"="Leer_Voltaje", "Message Queue"=w260) -> ("error out"=w259:errorcluster)  [unwired: 7 in, 1 out]
      }
      frame "Leer_Voltaje" {
        n121 = Flush Queue(queue=w270, error in (no error)=w274) -> (queue out=w275:refnum<queue>, error out=w276:errorcluster)  [unwired: 1 out]
        n122 = Unbundle By Name(w273) -> ("Inst_Keithley2002"=w279:refnum<queue>)
        n123 = call-poly "Enqueue Message.vi"("error in (no error)"=w276, "Message"="Leer_Frecuencia", "Message Queue"=w275) -> ("error out"=w282:errorcluster)  [unwired: 7 in, 1 out]
        n124 = call-poly "Enqueue Message.vi"("error in (no error)"=w282, "Message"="Leer_Instrumento", "Message Queue"=w279) -> ("error out"=w280:errorcluster)  [unwired: 7 in, 1 out]
        n125 = call "Time Delay2"("error in (no error)"=w280, "Delay Time (s)"=1.0) -> ("error out"=w272:errorcluster)  [unwired: 9 in]
      }
      frame "Leer_Frecuencia" {
        n126 = Flush Queue(queue=w284, error in (no error)=w287) -> (queue out=w288:refnum<queue>, error out=w289:errorcluster)  [unwired: 1 out]
        n127 = Unbundle By Name(w285) -> ("Inst_CNT90"=w292:refnum<queue>)
        n128 = call-poly "Enqueue Message.vi"("error in (no error)"=w289, "Message"="Leer_Indicadores", "Message Queue"=w288) -> ("error out"=w295:errorcluster)  [unwired: 7 in, 1 out]
        n129 = call-poly "Enqueue Message.vi"("error in (no error)"=w295, "Message"="Leer_Instrumento", "Message Queue"=w292) -> ("error out"=w293:errorcluster)  [unwired: 7 in, 1 out]
        n130 = call "Time Delay3"("error in (no error)"=w293, "Delay Time (s)"=1.0) -> ("error out"=w286:errorcluster)  [unwired: 9 in]
      }
      frame "Leer_Indicadores" {
        n131 = Flush Queue(queue=w307, error in (no error)=w308) -> (queue out=w309:refnum<queue>, error out=w310:errorcluster)  [unwired: 1 out]
        n132 = Unbundle By Name(w300) -> ("voltaje1"=w299:refnum<vi>, "frecuencia1"=w298:refnum<vi>)
        n133 = property class="DigNum (strict)"(reference=w299) -> ("Value"=w296:dbl)  [unwired: 1 in, 2 out]
        "voltaje2" <- w296
        "voltaje1" <- w296
        n134 = property class="DigNum (strict)"(reference=w298) -> ("Value"=→"frecuencia2" →"frecuencia1":dbl)  [unwired: 1 in, 2 out]
        n135 = call-poly "Enqueue Message.vi"("error in (no error)"=w310, "Message"="Leer_Voltaje", "Message Queue"=w309) -> ("error out"=w313:errorcluster)  [unwired: 7 in, 1 out]
        n136 = Less Or Equal?(x=w296, y=30.0) -> (x <= y?=w304:bool)
        n137 = Select(t=nan, s=w304, f=w296) -> (s? t:f=w302:dbl)
        n138 = Bundle By Name(cluster=w300, "voltMedido"=w302) -> (w301:refnum<class "Prueba07.lvclass">)
        n139 = call "Time Delay4"("error in (no error)"=w313, "Delay Time (s)"=1.0) -> ("error out"=w306:errorcluster)  [unwired: 9 in]
      }
      frame "EnviarVoltajeGEN" {
        n140 = Flush Queue(queue=w320, error in (no error)=w321) -> (queue out=w322:refnum<queue>, error out=w325:errorcluster)  [unwired: 1 out]
        n141 = Unbundle By Name(w319) -> ("Inst_DS360"=w329:refnum<queue>, "Inst_Keithley2002"=w334:refnum<queue>)
        n142 = Variant To Data(error in=w325, type=0.0, Variant=w317) -> (data=w327:dbl, error out=w332:errorcluster)
        n143 = call "Time Delay6"("error in (no error)"=w332, "Delay Time (s)"=0.5) -> ("error out"=w315:errorcluster)  [unwired: 9 in]
        n144 = call-poly "Enqueue Message.vi"("error in (no error)"=w315, "Message Data"=w327, "Message"="ActualizarVoltaje", "Message Queue"=w334) -> ("error out"=w330:errorcluster)  [unwired: 6 in, 1 out]
        n145 = call "Time Delay5"("error in (no error)"=w330, "Delay Time (s)"=0.5) -> ("error out"=w324:errorcluster)  [unwired: 9 in]
        n146 = local read "generar1"() -> (w316:bool)
        n147 = call-poly "Enqueue Message.vi"("error in (no error)"=w324, "Message Data"=w327, "Message"="ActualizarAmplitud", "Message Queue"=w329) -> ("error out"=w326:errorcluster)  [unwired: 6 in, 1 out]
        n148 = case shown="True" w316 {
          tunnel: w326 -> [w336 w340]
          tunnel: [w336 w339] -> w318
          tunnel: w322 -> [_ w338]
          frame False {
          }
          frame True {
            n149 = call-poly "Enqueue Message.vi"("error in (no error)"=w340, "Message"="Leer_Voltaje", "Message Queue"=w338) -> ("error out"=w339:errorcluster)  [unwired: 7 in, 1 out]
          }
        }
      }
      frame "EnviarVoltajeGEN_2" {
        n150 = Unbundle By Name(w345) -> ("Inst_DS360"=w351:refnum<queue>, "Inst_Keithley2002"=w356:refnum<queue>)
        n151 = Variant To Data(error in=w348, type=0.0, Variant=w343) -> (data=w349:dbl, error out=w354:errorcluster)
        n152 = call "Time Delay9"("error in (no error)"=w354, "Delay Time (s)"=0.5) -> ("error out"=w342:errorcluster)  [unwired: 9 in]
        n153 = call-poly "Enqueue Message.vi"("error in (no error)"=w342, "Message Data"=w349, "Message"="ActualizarVoltaje", "Message Queue"=w356) -> ("error out"=w352:errorcluster)  [unwired: 6 in, 1 out]
        n154 = call "Time Delay8"("error in (no error)"=w352, "Delay Time (s)"=0.5) -> ("error out"=w347:errorcluster)  [unwired: 9 in]
        n155 = call-poly "Enqueue Message.vi"("error in (no error)"=w347, "Message Data"=w349, "Message"="ActualizarAmplitud", "Message Queue"=w351) -> ("error out"=w344:errorcluster)  [unwired: 6 in, 1 out]
      }
      frame "EnviarVoltajeGEN_3" {
        n156 = Unbundle By Name(w362) -> ("Inst_DS360"=w368:refnum<queue>, "Inst_Keithley2002"=w373:refnum<queue>)
        n157 = Variant To Data(error in=w365, type=0.0, Variant=w360) -> (data=w366:dbl, error out=w371:errorcluster)
        n158 = call "Time Delay13"("error in (no error)"=w371, "Delay Time (s)"=0.5) -> ("error out"=w359:errorcluster)  [unwired: 9 in]
        n159 = call-poly "Enqueue Message.vi"("error in (no error)"=w359, "Message Data"=w366, "Message"="ActualizarVoltaje", "Message Queue"=w373) -> ("error out"=w369:errorcluster)  [unwired: 6 in, 1 out]
        n160 = call "Time Delay12"("error in (no error)"=w369, "Delay Time (s)"=0.5) -> ("error out"=w364:errorcluster)  [unwired: 9 in]
        n161 = call-poly "Enqueue Message.vi"("error in (no error)"=w364, "Message Data"=w366, "Message"="ActualizarAmplitud", "Message Queue"=w368) -> ("error out"=w361:errorcluster)  [unwired: 6 in, 1 out]
      }
      frame "FrecAmp2_Vref" {
        # "Vref guardado anterioemente"
        n162 = Flush Queue(queue=w393, error in (no error)=w396) -> (queue out=w392:refnum<queue>, error out=w394:errorcluster)  [unwired: 1 out]
        n163 = Unbundle By Name(w381) -> ("Control references"=w379:T7)
        n164 = call "_get control reference by name.vi"("error in (no error)"=w394, "Control name"="generarNivMax", "Control references"=w379) -> ("error out"=w380:errorcluster, "Ctl Refnum"=w376:refnum<vi>)  [unwired: 3 in]
        n165 = Build Array(w376) -> (w375:refnum<vi>[])
        n166 = call "Enable_Visible Buttons.vi"("Enable? (T)"=FALSE, "Controls Ref Array"=w375) -> ()  [unwired: 10 in]
        n167 = local read "Vref"() -> (w390:dbl)
        n168 = local write "GEN"("NivRef" ("GEN")) -> ()
        n169 = Divide(x=w390, y=1000.0) -> (x/y=w382:dbl)
        n170 = call-poly "Enqueue Message.vi"("error in (no error)"=w380, "Message"="updateUI", "Message Queue"=w392) -> ("error out"=w395:errorcluster, "dup Message Queue"=w386:refnum<queue>)  [unwired: 7 in]
        n171 = Bundle By Name(cluster=w381, "amp"=w382) -> (w391:refnum<class "Prueba07.lvclass">)
        n172 = call-poly "Enqueue Message.vi"("Message Data"=w382, "Message"="EnviarVoltajeGEN_2", "Message Queue"=w386) -> ("dup Message Queue"=w384:refnum<queue>)  [unwired: 7 in, 1 out]
        n173 = call-poly "Enqueue Message.vi"("Message"="iniciarGEN_2", "Message Queue"=w384) -> ()  [unwired: 8 in, 2 out]
      }
      frame "FrecAmp2_Vref_NivMax" {
        n174 = Flush Queue(queue=w424, error in (no error)=w425) -> (queue out=w423:refnum<queue>, error out=w398:errorcluster)  [unwired: 1 out]
        n175 = Unbundle By Name(w399) -> ("Control references"=w404:T7)
        n176 = call "_get control reference by name.vi"("error in (no error)"=w398, "Control name"="generarNivRef", "Control references"=w404) -> ("error out"=w397:errorcluster, "Ctl Refnum"=w401:refnum<vi>)  [unwired: 3 in]
        n177 = call "FGV_fila_2.vi"("action"=enum16{"increment", "set_start", "get"}."get") -> ("fila out"=w419:i32)  [unwired: 3 in, 1 out]
        n178 = Build Array(w401) -> (w400:refnum<vi>[])
        n179 = local read "Vref_NivMax"() -> (w421:dbl[])
        n180 = call "Enable_Visible Buttons.vi"("Enable? (T)"=FALSE, "Controls Ref Array"=w400) -> ()  [unwired: 10 in]
        n181 = Subtract(x=w419, y=11) -> (x-y=w417:i32)
        n182 = local write "GEN"("RefNivMax" ("GEN")) -> ()
        n183 = Index Array(array=w421, index=w417) -> (element=w416:dbl)
        n184 = call-poly "Enqueue Message.vi"("error in (no error)"=w397, "Message"="updateUI", "Message Queue"=w423) -> ("error out"=w412:errorcluster, "dup Message Queue"=w410:refnum<queue>)  [unwired: 7 in]
        n185 = Divide(x=w416, y=1000.0) -> (x/y=w405:dbl)
        n186 = Bundle By Name(cluster=w399, "amp"=w405) -> (w422:refnum<class "Prueba07.lvclass">)
        n187 = call-poly "Enqueue Message.vi"("error in (no error)"=w412, "Message Data"=w405, "Message"="EnviarVoltajeGEN_3", "Message Queue"=w410) -> ("error out"=w411:errorcluster, "dup Message Queue"=w409:refnum<queue>)  [unwired: 6 in]
        n188 = call-poly "Enqueue Message.vi"("error in (no error)"=w411, "Message"="iniciarGEN_3", "Message Queue"=w409) -> ("error out"=w408:errorcluster)  [unwired: 7 in, 1 out]
      }
      frame "guardarMedicionesNivRef" {
        w446 = 1  # col
        # "Actualiza el nuevo valor\nde Referencia dB en Combo Box"
        # "Guarda el Valor medido en DMM\nen la Tabla"
        n189 = Flush Queue(queue=w451, error in (no error)=w452) -> (queue out=w450:refnum<queue>, error out=w449:errorcluster)  [unwired: 1 out]
        n190 = Unbundle By Name(w428) -> ("Tabla"=w443:string[][], "voltMedido"=w444:dbl)
        n191 = Unbundle By Name(w428) -> ("Control references"=w433:T7)
        n192 = call "FGV_fila.vi"("action"=enum16{"increment", "set_start", "get"}."get") -> ("error out"=w439:errorcluster, "fila out"=w440:i32)  [unwired: 3 in]
        n193 = call-poly "Enqueue Message.vi"("error in (no error)"=w449, "Message"="detenerGEN", "Message Queue"=w450) -> ("error out"=w427:errorcluster)  [unwired: 7 in, 1 out]
        n194 = call "escribeEnTablaUnValor.vi"("element"=w444, "fila"=w440, "col"=w446, "tabla in"=w443) -> ("tabla out"=w445:string[][])  [unwired: 7 in]
        n195 = call "_get control reference by name.vi"("error in (no error)"=w427, "Control name"="generarNivMax", "Control references"=w433) -> ("error out"=w426:errorcluster, "Ctl Refnum"=w430:refnum<vi>)  [unwired: 3 in]
        n196 = Build Array(w430) -> (w429:refnum<vi>[])
        n197 = local read "n°filas"() -> (w436:i32)
        n198 = Bundle By Name(cluster=w428, "Tabla"=w445) -> (w447:refnum<class "Prueba07.lvclass">)
        n199 = call "FGV_fila.vi"("error in (no error)"=w439, "action"=enum16{"increment", "set_start", "get"}."increment") -> ("fila out"=w438:i32)  [unwired: 2 in, 1 out]
        n200 = call "Enable_Visible Buttons.vi"("Enable? (T)"=TRUE, "Controls Ref Array"=w429) -> ()  [unwired: 10 in]
        n201 = Decrement(x=w436) -> (x-1=w437:i32)
        n202 = Greater?(x=w438, y=w437) -> (0:w435:bool)
        n203 = Unbundle By Name(w447) -> ("Tabla"=w448:string[][])
        n204 = case shown="True" w435 {
          frame False {
          }
          frame True {
            n205 = call "FGV_fila.vi"("fila_inicial"=0, "action"=enum16{"increment", "set_start", "get"}."set_start") -> ()  [unwired: 2 in, 2 out]
            n206 = One Button Dialog(message="Llegamos al final del rango") -> ()  [unwired: 1 in, 1 out]
          }
        }
        n207 = local write "Tabla"(w448) -> ()
      }
      frame "guardarMedicionesNivMax" {
        w478 = 1  # col
        # "Actualiza el nuevo valor\nde Referencia dB en Combo Box"
        # "Guarda el Valor medido en DMM\nen la Tabla"
        n208 = Flush Queue(queue=w483, error in (no error)=w484) -> (queue out=w482:refnum<queue>, error out=w481:errorcluster)  [unwired: 1 out]
        n209 = Unbundle By Name(w457) -> ("Tabla"=w475:string[][], "voltMedido"=w476:dbl)
        n210 = Unbundle By Name(w457) -> ("Control references"=w456:T7)
        n211 = call "FGV_fila_2.vi"("action"=enum16{"increment", "set_start", "get"}."get") -> ("error out"=w471:errorcluster, "fila out"=w472:i32)  [unwired: 3 in]
        n212 = call-poly "Enqueue Message.vi"("error in (no error)"=w481, "Message"="detenerGEN", "Message Queue"=w482) -> ("error out"=w459:errorcluster)  [unwired: 7 in, 1 out]
        n213 = call "escribeEnTablaUnValor.vi"("element"=w476, "fila"=w472, "col"=w478, "tabla in"=w475) -> ("tabla out"=w477:string[][])  [unwired: 7 in]
        n214 = local read "n°filas"() -> (w467:i32)
        n215 = call "_get control reference by name.vi"("error in (no error)"=w459, "Control name"="generarNivRef", "Control references"=w456) -> ("error out"=w458:errorcluster, "Ctl Refnum"=w461:refnum<vi>)  [unwired: 3 in]
        n216 = Bundle By Name(cluster=w457, "Tabla"=w477) -> (w479:refnum<class "Prueba07.lvclass">)
        n217 = Build Array(w461) -> (w460:refnum<vi>[])
        n218 = Add(x=w467, y=11) -> (x+y=w465:i32)
        n219 = call "FGV_fila_2.vi"("error in (no error)"=w471, "action"=enum16{"increment", "set_start", "get"}."increment") -> ("fila out"=w470:i32)  [unwired: 2 in, 1 out]
        n220 = call "Enable_Visible Buttons.vi"("Enable? (T)"=TRUE, "Controls Ref Array"=w460) -> ()  [unwired: 10 in]
        n221 = Decrement(x=w465) -> (x-1=w469:i32)
        n222 = Greater?(x=w470, y=w469) -> (0:w468:bool)
        n223 = Unbundle By Name(w479) -> ("Tabla"=w480:string[][])
        n224 = case shown="True" w468 {
          frame False {
          }
          frame True {
            n225 = call "FGV_fila_2.vi"("fila_inicial"=11, "action"=enum16{"increment", "set_start", "get"}."set_start") -> ()  [unwired: 2 in, 2 out]
            n226 = One Button Dialog(message="Llegamos al final del rango") -> ()  [unwired: 1 in, 1 out]
          }
        }
        n227 = local write "Tabla"(w480) -> ()
      }
      frame "ingresaMediciones" {
        n228 = Flush Queue(queue=w496, error in (no error)=w501) -> (queue out=w495:refnum<queue>, error out=w497:errorcluster)  [unwired: 1 out]
        n229 = Variant To Data(error in=w497, type=string[][] [] ("NewVal"), Variant=w489) -> (data=w492:string[][], error out=w494:errorcluster)
        n230 = control-ref of="Tabla"() -> (w498:refnum<vi>)
        n231 = call "ingresaMediciones.vi"("error in (no error)"=w494, "Tbl Refnum"=w498, "New Value"=w492, "Prueba07 in"=w491) -> ("error out"=w500:errorcluster, "Prueba07 out"=w490:refnum<class "Prueba07.lvclass">)  [unwired: 6 in]
        n232 = call-poly "Enqueue Message.vi"("error in (no error)"=w500, "Message"="cumplimiento", "Message Queue"=w495) -> ("error out"=w499:errorcluster)  [unwired: 7 in, 1 out]
      }
      frame "cumplimiento" {
        (unwired) T8 {"Estados"=enum."listo_evaluar", "Data"=variant} ("element")
        n233 = call "cumplimiento.vi"("error in (no error)"=w508, "Prueba07 in"=w504) -> ("error out"=w507:errorcluster, "Prueba07 out"=w503:refnum<class "Prueba07.lvclass">)  [unwired: 8 in]
        n234 = call-poly "Enqueue Message.vi"("error in (no error)"=w507, "Message"="listo_evaluar", "Message Queue"=w505) -> ("error out"=w506:errorcluster)  [unwired: 7 in, 1 out]
      }
      frame "listo_evaluar" {
        n235 = Unbundle By Name(w520) -> ("Tabla"=w523:string[][])
        n236 = local read "n°filas"() -> (w511:i32)
        n237 = Unbundle By Name(w520) -> ("Tabla"=w524:string[][])
        n238 = local read "n°filas"() -> (w512:i32)
        n239 = Index Array(array=w523, index (col)=8 ("disabled index (col)")) -> (element=w516:string[])  [unwired: 1 in]
        n240 = Index Array(array=w524, index (col)=8 ("disabled index (col)")) -> (element=w519:string[])  [unwired: 1 in]
        n241 = Array Subset(array=w519, index=0, length=w512) -> (w517:string[])
        n242 = Array Subset(array=w516, index=11, length=w511) -> (w515:string[])
        n243 = for {
          tunnel: [w547] -> w522 mode=indexing
          tunnel: w515 -> [w545] mode=indexing
          n244 = Not Equal?(x=w545, y="--") -> (x != y?=w547:bool)
        }
        n245 = for {
          tunnel: [w550] -> w525 mode=indexing
          tunnel: w517 -> [w548] mode=indexing
          n246 = Not Equal?(x=w548, y="--") -> (x != y?=w550:bool)
        }
        n247 = And Array Elements(Boolean array=w522) -> (logical AND=w513:bool)
        n248 = And Array Elements(Boolean array=w525) -> (logical AND=w514:bool)
        n249 = And(x=w514, y=w513) -> (x .and. y?=w509:bool)
        n250 = case shown="True" w509 {
          tunnel: w529 -> [w533 w544]
          tunnel: [w532 w543] -> w528
          tunnel: w527 -> [w530 w542]
          frame False {
            n251 = local read "generarNivRef"() -> (w535:bool)
            n252 = local read "generarNivMax"() -> (w534:bool)
            n253 = Or(x=w535, y=w534) -> (x .or. y?=w531:bool)
            n254 = case shown="False" w531 {
              tunnel: w533 -> [w536 w540]
              tunnel: [w536 w539] -> w532
              tunnel: w530 -> [_ w538]
              frame False {
              }
              frame True {
                n255 = call-poly "Enqueue Message.vi"("error in (no error)"=w540, "Message"="Leer_Voltaje", "Message Queue"=w538) -> ("error out"=w539:errorcluster)  [unwired: 7 in, 1 out]
              }
            }
          }
          frame True {
            n256 = call-poly "Enqueue Message.vi"("error in (no error)"=w544, "Message"="evaluar", "Message Queue"=w542) -> ("error out"=w543:errorcluster)  [unwired: 7 in, 1 out]
          }
        }
      }
      frame "evaluar" {
        # "si todos cumplen\nentonces el ensayo\ncumple"
        n257 = Unbundle By Name(w563) -> ("Tabla"=w567:string[][])
        n258 = Unbundle By Name(w563) -> ("Tabla"=w566:string[][])
        n259 = local read "n°filas"() -> (w555:i32)
        n260 = local read "n°filas"() -> (w554:i32)
        n261 = call-poly "Enqueue Message.vi"("error in (no error)"=w570, "Message"="final", "Message Queue"=w569) -> ("error out"=w568:errorcluster)  [unwired: 7 in, 1 out]
        n262 = Index Array(array=w567, index (col)=8 ("disabled index (col)")) -> (element=w558:string[])  [unwired: 1 in]
        n263 = Index Array(array=w566, index (col)=8 ("disabled index (col)")) -> (element=w557:string[])  [unwired: 1 in]
        n264 = Array Subset(array=w557, index=11, length=w554) -> (w552:string[])
        n265 = Array Subset(array=w558, index=0, length=w555) -> (w553:string[])
        n266 = for {
          tunnel: [w578] -> w572 mode=indexing
          tunnel: w553 -> [w576] mode=indexing
          n267 = Equal?(x=w576, y="Cumple") -> (x = y?=w578:bool)
        }
        n268 = for {
          tunnel: [w575] -> w564 mode=indexing
          tunnel: w552 -> [w573] mode=indexing
          n269 = Equal?(x=w573, y="Cumple") -> (x = y?=w575:bool)
        }
        n270 = And Array Elements(Boolean array=w572) -> (logical AND=w561:bool)
        n271 = And Array Elements(Boolean array=w564) -> (logical AND=w560:bool)
        n272 = And(x=w561, y=w560) -> (x .and. y?=→"cumple_no_cumple":bool)
      }
      frame "final" {
        n273 = local read "cumple_no_cumple"() -> (w581:bool)
        "cumple" <- w581
        n274 = Not(x=w581) -> (.not. x?=→"no_cumple":bool)
        n275 = Select(t="Cumple", s=w581, f="No Cumple") -> (s? t:f=→"resultado":string)
      }
      frame "updateUI" {
        n276 = local read "GEN"() -> (w588:string)
        n277 = case shown="\"NivRef\", Default" w588 {
          tunnel: enum16{"increment", "set_start", "get"}."get" ("action") -> [w597 w599]
          tunnel: [w596 w598] -> w589
          frame "RefNivMax" {
            n278 = call "FGV_fila_2.vi"("action"=w597) -> ("fila out"=w596:i32)  [unwired: 3 in, 1 out]
          }
          frame "NivRef", Default {
            n279 = call "FGV_fila.vi"("action"=w599) -> ("fila out"=w598:i32)  [unwired: 3 in, 1 out]
          }
        }
        n280 = Unbundle By Name(w594) -> ("Tabla"=w593:string[][])
        n281 = Index Array(array=w593, index (row) #1=w589, index (col) #1=0 ("disabled index (col)"), index (row) #2=w589, index (col) #2=2 ("index (col)")) -> (element #1=→"RangoRefActual":string, element #2=→"RefActual":string)
      }
      frame "DatoRecibidoCNT90" {
        n282 = Variant To Data(error in=w604, type=0.0 ("y"), Variant=w602) -> (error out=w601:errorcluster)  [unwired: 1 out]
      }
      frame "DatoRecibidoK2002" {
        n283 = Variant To Data(error in=w609, type=0.0 ("y"), Variant=w607) -> (error out=w606:errorcluster)  [unwired: 1 out]
      }
      frame "detenerGEN" {
        w628 = 0.0 ("voltaje1")
        n284 = Flush Queue(queue=w616, error in (no error)=w617) -> (error out=w611:errorcluster)  [unwired: 2 out]
        n285 = Unbundle By Name(w615) -> ("Inst_DS360"=w621:refnum<queue>)
        n286 = call "Time Delay14"("error in (no error)"=w611, "Delay Time (s)"=0.5) -> ("error out"=w610:errorcluster)  [unwired: 9 in]
        n287 = local write "voltaje1"(w628) -> ()
        n288 = local write "voltaje2"(w628) -> ()
        n289 = local write "frecuencia1"(w628) -> ()
        n290 = local write "frecuencia2"(w628) -> ()
        n291 = call-poly "Enqueue Message.vi"("error in (no error)"=w610, "Message"="Deshabilitar_Generador", "Message Queue"=w621) -> ("error out"=w620:errorcluster)  [unwired: 7 in, 1 out]
        n292 = call "Time Delay7"("error in (no error)"=w620, "Delay Time (s)"=0.5) -> ("error out"=w619:errorcluster)  [unwired: 9 in]
        n293 = Unbundle By Name(w613) -> ("Control references"=w623:T7)
        n294 = call-poly "get control reference by name.vi"("error in (no error)"=w619, "Control name"="guardar_Vref" ("String"), "Control references"=w623) -> ("error out"=w614:errorcluster, "Ctl Refnum"=w625:refnum<vi>)  [unwired: 3 in]
        n295 = Build Array(w625) -> (w624:refnum<vi>[])
        n296 = call "Enable_Visible Buttons.vi"("Enable? (T)"=FALSE, "Controls Ref Array"=w624) -> ()  [unwired: 10 in]
      }
      frame "guardarVref" {
        n297 = flat-sequence {
          tunnel: w630 -> [w634]
          tunnel: [w634] -> w629
          frame #0 {
            n298 = local read "AjusteAmp"() -> (w635:T1)
            "Vref" <- w635
            n299 = Number To Fractional String(number=w635, precision (6)=i16 3) -> (F-format string=w636:string)  [unwired: 2 in]
            n300 = Format Into String(format string="Se guardó Vref = %s mV", w636) -> (resulting string=w639:string)  [unwired: 2 in, 1 out]
            n301 = One Button Dialog(message=w639) -> ()  [unwired: 1 in, 1 out]
          }
        }
        n302 = property on="seguir" class="Bool"(error in=w629, "DisabledEnum"=T6."Enabled" ("Disabled")) -> (error out=w631:errorcluster)  [unwired: 1 in, 1 out]
      }
      frame "DetieneInstrumentos" {
      }
      frame "Exit" {
        w643 = TRUE
        # "#evangelio Manda a cerrar el EHL"
        # "#evangelio Manda a cerrar todos los Loops"
        n303 = Release Queue(queue=w648, error in (no error)=w649) -> (error out=w653:errorcluster)  [unwired: 1 in, 2 out]
        n304 = Unbundle By Name(w644) -> ("Control references"=w654:T7)
        n305 = for {
          tunnel: w647 -> [w657] mode=indexing
          tunnel: w645 -> [w656]
          tunnel: TRUE -> [w655]
          n306 = call-poly "Enqueue Message.vi"("Priority Message? (F)"=w655, "Message"=w656, "Message Queue"=w657) -> ()  [unwired: 7 in, 2 out]
        }
        n307 = call "Close All Ref.vi"("error in (no error)"=w653, "Control references"=w654) -> ("error out"=w651:errorcluster)  [unwired: 9 in]
        n308 = call "Fire User Event - Stop.vi"("error in (no error)"=w651, "Event Data"=w643, "User Event"="Exit EHL", "User Event in"=w646) -> ("error out"=w642:errorcluster)  [unwired: 7 in]
      }
      frame "Confirmar Salida" {
        n309 = Two Button Dialog(message="¿Quieres cerrar la aplicación?", 1:"No" ("T button name (\"OK\")"), 2:"Si" ("T button name (\"OK\")")) -> (T button?=w662:bool)
        n310 = case shown="True" w662 {
          tunnel: w661 -> [w666 w669]
          tunnel: [w666 w673] -> w659
          tunnel: w660 -> [_ w671]
          frame False {
          }
          frame True {
            n311 = call-poly "Enqueue Message.vi"("error in (no error)"=w669, "Message"="Detener_Instrumento", "Message Queue"=w671) -> ("error out"=w668:errorcluster, "dup Message Queue"=w670:refnum<queue>)  [unwired: 7 in]
            n312 = call-poly "Enqueue Message.vi"("error in (no error)"=w668, "Message"="Exit", "Message Queue"=w670) -> ("error out"=w673:errorcluster)  [unwired: 7 in, 1 out]
          }
        }
      }
      frame Default {
        n313 = xnode "Error Ring"("parameter 0"=w676) -> ("error out"=w675:errorcluster)
      }
      frame "Error" {
        w688 = T10 1 items=["no dialog", "OK message", "continue or stop message", "OK message + warnings", "continue/stop + warnings"] ("type of dialog (OK msg:1)")
        n314 = Variant To Data(error in=w692, type=errorcluster {"status"=FALSE, "code"=0, "source"=""} ("error out"), Variant=w687) -> (data=w685:errorcluster, error out=w684:errorcluster)
        n315 = call <vilib>:"Simple Error Handler.vi"("type of dialog (OK msg:1)"=w688, "error in (no error)"=w685) -> ()  [unwired: 3 in, 5 out]
        n316 = call-poly "Enqueue Message.vi"("error in (no error)"=w684, "Message"="Exit", "Message Queue"=w691) -> ("error out"=w690:errorcluster)  [unwired: 7 in, 1 out]
      }
      frame "----------------------Controles----------------------" {
      }
    }
    n317 = call "Error Handler - Message Handling Loop.vi"("error in (no error)"=w101, "Message Queue"=w99) -> ("dup error in"=w100:errorcluster)  [unwired: 8 in, 1 out]
    n318 = Unbundle By Name(w111) -> ("Tabla"=w110:string[][])
    n319 = local write "Tabla"(w110) -> ()
  }
  n320 = call "Inst_K2002.vi"("All Message Queues in"=w5, "Prueba31 in"=w6) -> ()  [unwired: 9 in, 1 out]
  n321 = call "Inst_DS360.vi"("All Message Queues in"=w5, "Prueba07 in"=w6) -> ()  [unwired: 9 in, 1 out]
  n322 = call "Inst_CNT90.vi"("All Message Queues in"=w5, "Prueba31 in"=w6) -> ()  [unwired: 9 in, 1 out]
  n323 = call-dynamic "CleanUp.vi"("Prueba07 in"=w2) -> ("Prueba07 out"=→"Prueba07 out":refnum<class "Prueba07.lvclass">)  [unwired: 9 in, 1 out]
  n324 = Merge Errors(w21, w20) -> (→"error out":errorcluster)
